vi "process_stream_data.vi"(7 "Queues":T1, 8 "error in (no error)":errorcluster, 10 "aData Out":dbl[][](array[numeric]), 11 "Loop Data In":T3[](array[typedef])) -> (0 "error out":errorcluster, 3 "Loop Data Out":T3[](array[typedef]))   [LabVIEW 2025, in "LabJackEKG.lvlib"]
uses:
  LabJackEKG.lvlib
  Tests/StreamProducerLoopData.ctl
  Typedefs/LabJackGlobalResources.ctl
  Typedefs/CounterQueues.ctl
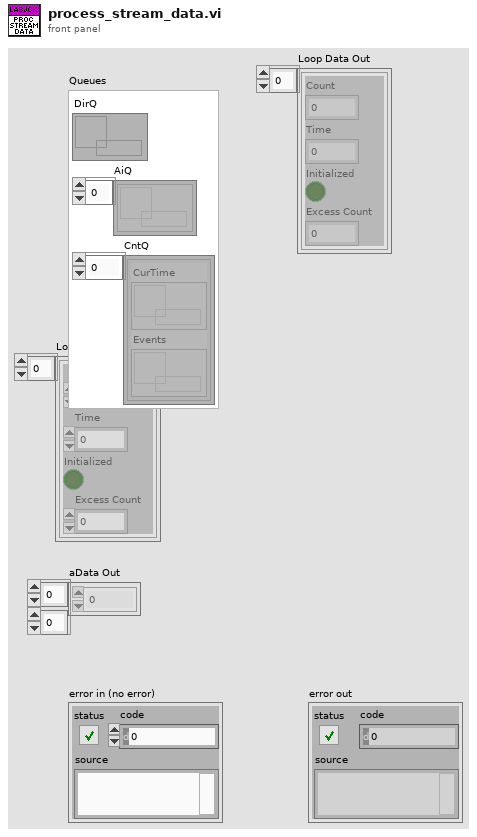
[diagram p1: front panel]
types:
  T1 = typedef "LabJackEKG.lvlib/LabJackGlobalResources.ctl" = cluster{"DirQ":refnum<queue>, "AiQ":refnum<queue>[], "CntQ":T2[]}
  T2 = typedef "LabJackEKG.lvlib/CounterQueues.ctl" = cluster{"CurTime":refnum<queue>, "Events":refnum<queue>}
  T3 = typedef "LabJackEKG.lvlib/StreamProducerLoopData.ctl" = cluster{"Count":i64, "Time":dbl, "Initialized":bool, "Excess Count":i64}
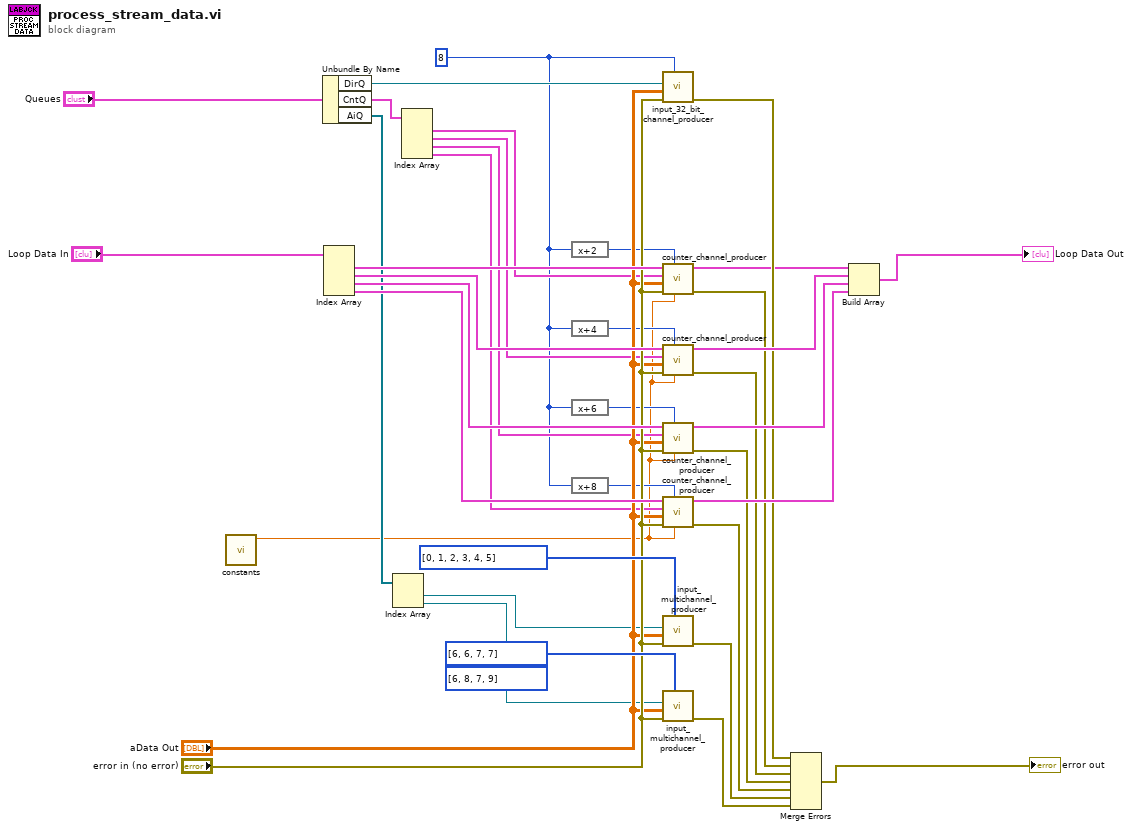
[diagram p0: block diagram]
diagram:
  (unwired) i32[] [6, 8, 7, 9] ("Indices")
  w2 = 8 ("Channel")
  n1 = call "constants.vi"() -> ("Sampling Frequency [Hz]"=w1:dbl)  [unwired: 10 in, 1 out]
  n2 = Unbundle By Name("Queues") -> ("DirQ"=w7:refnum<queue>, "CntQ"=w28:T2[], "AiQ"=w29:refnum<queue>[])
  n3 = Index Array(array="Loop Data In") -> (element #1=w35:T3, element #2=w36:T3, element #3=w37:T3, element #4=w38:T3)  [unwired: 4 in]
  n4 = Index Array(array=w29) -> (element #1=w19:refnum<queue>, element #2=w20:refnum<queue>)  [unwired: 2 in]
  n5 = Index Array(array=w28) -> (element #1=w13:T2, element #2=w14:T2, element #3=w15:T2, element #4=w16:T2)  [unwired: 4 in]
  n6 = expression code="x+2"(w2) -> (w6:i32)
  n7 = expression code="x+4"(w2) -> (w5:i32)
  n8 = expression code="x+6"(w2) -> (w4:i32)
  n9 = expression code="x+8"(w2) -> (w3:i32)
  n10 = call "input_32_bit_channel_producer.vi"("Index"=w2, "error in (no error)"="error in (no error)", "aData Out"="aData Out", "DirQ"=w7) -> ("error out"=w24:errorcluster)  [unwired: 7 in]
  n11 = call "counter_channel_producer.vi"("Sampling Frequency [Hz]"=w1, "Channel"=w6, "error in (no error)"="error in (no error)", "aData Out"="aData Out", "Queue in"=w13, "output cluster in"=w35) -> ("error out"=w8:errorcluster, "output cluster out"=w9:T3)  [unwired: 4 in]
  n12 = call "counter_channel_producer.vi"("Sampling Frequency [Hz]"=w1, "Channel"=w5, "error in (no error)"="error in (no error)", "aData Out"="aData Out", "Queue in"=w14, "output cluster in"=w36) -> ("error out"=w10:errorcluster, "output cluster out"=w30:T3)  [unwired: 4 in]
  n13 = call "counter_channel_producer.vi"("Sampling Frequency [Hz]"=w1, "Channel"=w4, "error in (no error)"="error in (no error)", "aData Out"="aData Out", "Queue in"=w15, "output cluster in"=w37) -> ("error out"=w12:errorcluster, "output cluster out"=w31:T3)  [unwired: 4 in]
  n14 = call "counter_channel_producer.vi"("Sampling Frequency [Hz]"=w1, "Channel"=w3, "error in (no error)"="error in (no error)", "aData Out"="aData Out", "Queue in"=w16, "output cluster in"=w38) -> ("error out"=w11:errorcluster, "output cluster out"=w32:T3)  [unwired: 4 in]
  n15 = call "input_multichannel_producer.vi"("Indices"=i32[] [0, 1, 2, 3, 4, 5], "error in (no error)"="error in (no error)", "aData Out"="aData Out", "Q"=w19) -> ("error out"=w18:errorcluster)  [unwired: 7 in]
  n16 = call "input_multichannel_producer.vi"("Indices"=i32[] [6, 6, 7, 7], "error in (no error)"="error in (no error)", "aData Out"="aData Out", "Q"=w20) -> ("error out"=w21:errorcluster)  [unwired: 7 in]
  n17 = Merge Errors(w24, w8, w10, w12, w11, w18, w21) -> (→"error out":errorcluster)
  n18 = Build Array(w9, w30, w31, w32) -> (→"Loop Data Out":T3[])
